vi "MessageEvent.vi"(0 "reference in":refnum<class "DP_WebView.lvclass">, 5 "error in (no error)":errorcluster) -> (14 "reference out":refnum<class "DP_WebView.lvclass">, 15 "Event Callback":refnum<k27>, 16 "WebMessageAsJson":refnum<user-event>, 19 "error out":errorcluster)   [LabVIEW 2020, in "DP_WebView.lvclass"]
uses:
  DP_WebView.lvclass
  CallBackVIs/Callback_WebMessage.vi
  C:/Projects/DependencyViewer/DependencyViewer/DP_WebView_class/data/Microsoft.Web.WebView2.Core.dll
  data/Microsoft.Web.WebView2.Core.dll
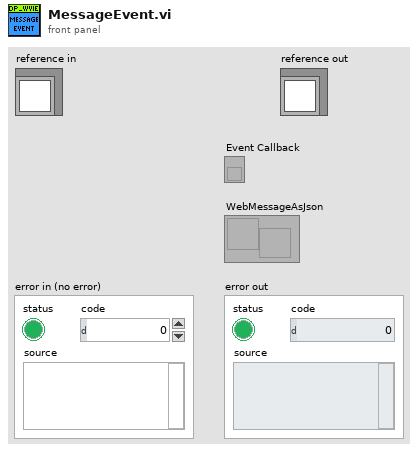
[diagram p1: front panel]
types:
  T1 = typedef "DP_WebView.lvclass/ObjectAttributes.ctl" = cluster{"WebView Container":refnum<k24>, "CoreWebViewRef":refnum<k24>, "Status":i32, "Status Message":string, "User Data Folder":path, "BrowserProcessId":u32}
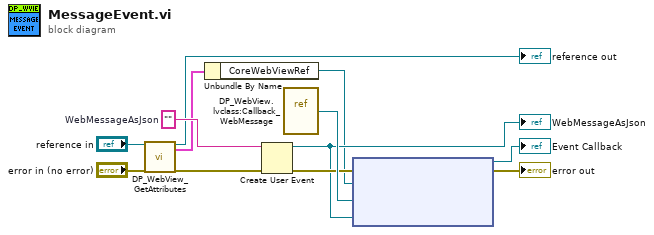
[diagram p0: block diagram]
diagram:
  w12 = ""  # WebMessageAsJson
  n1 = call "DP_WebView_GetAttributes.vi"("reference in"="reference in", "error in (no error)"="error in (no error)") -> ("reference out"=→"reference out":refnum<class "DP_WebView.lvclass">, "Data"=w3:T1, "error out"=w9:errorcluster)  [unwired: 14 in, 1 out]
  n2 = Unbundle By Name(w3) -> ("CoreWebViewRef"=w4:refnum<k24>)
  n3 = Create User Event(user event datatype=w12, error in=w9) -> (user event=w5:refnum<user-event>, error out=w10:errorcluster)
  "WebMessageAsJson" <- w5
  n4 = vi-ref "DP_WebView.lvclass:Callback_WebMessage.vi"() -> ("vi reference"=w11:refnum<vi>)
  n5 = node(w10, w4, w11, w5) -> (→"Event Callback":refnum<k27>, →"error out":errorcluster)  [unwired: 1 in]
